vi "Create Fixed Length String.vi"(1 "String":string="test", 2 "Length":u32=15) -> (0 "String out":string="test           ")   [LabVIEW 2018, in "Protocol Interface.lvlib" / "Protocol Interface.lvclass"]
uses:
  Protocol Interface.lvclass
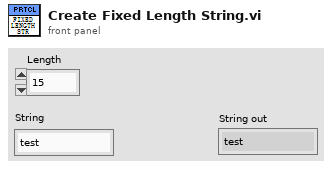
[diagram p1: front panel]
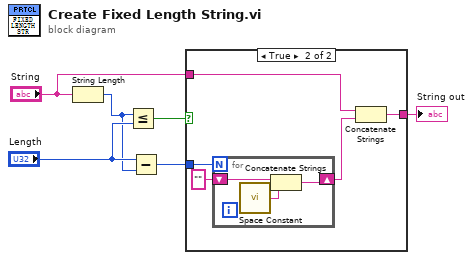
[diagram p0: block diagram]
diagram:
  n1 = String Length(string="String") -> (length=w4:i32)
  n2 = Less Or Equal?(x=w4, y="Length") -> (x <= y?=w6:bool)
  n3 = Subtract(x="Length", y=w4) -> (x-y=w3:u32)
  n4 = case shown="True" w6 {
    tunnel: w3 -> [_ w12]
    tunnel: "String" -> [w7 w10]
    tunnel: [w7 w8] -> w1
    frame False {
    }
    frame True {
      n5 = for {
        N: w12 -> [_]
        shift-right: [w13] -> w9
        shift-left: "" -> [w14]
        n6 = call <vilib>:"Space Constant.vi"() -> ("String"=w15:string)
        n7 = Concatenate Strings(w14, w15) -> (w13:string)
      }
      n8 = Concatenate Strings(w10, w9) -> (w8:string)
    }
  }
  "String out" <- w1
